vi "guadagno.vi"() -> ()   [LabVIEW 2014]
uses:
  <vilib>/measure/maspectr.llb/FFT Power Spectrum and PSD for N Chan.vi
  <vilib>/measure/mascope.llb/Amplitude and Levels N chan.vi
  <vilib>/measure/NI_MABase.lvlib
  <vilib>/measure/NI_MAPro.lvlib
panel:
  out "x/y 2":T1(array[cluster])
  out "Waveform Graph 4":cluster{"f0":dbl, "df":dbl, "magnitude":dbl[]}[](graph)
  out "x/y":dbl[](array[numeric])
  out "Waveform Graph 3":dynamicdata(graph)
  out "Waveform Graph 2":dynamicdata(graph)
  out "Waveform Graph":waveform(dbl)(graph)
  in  "signal type":T2(ring)
  in  "amplitude":dbl=1.0 format="%0.2p"
  in  "frequency":dbl=10.0 format="%#_13g"
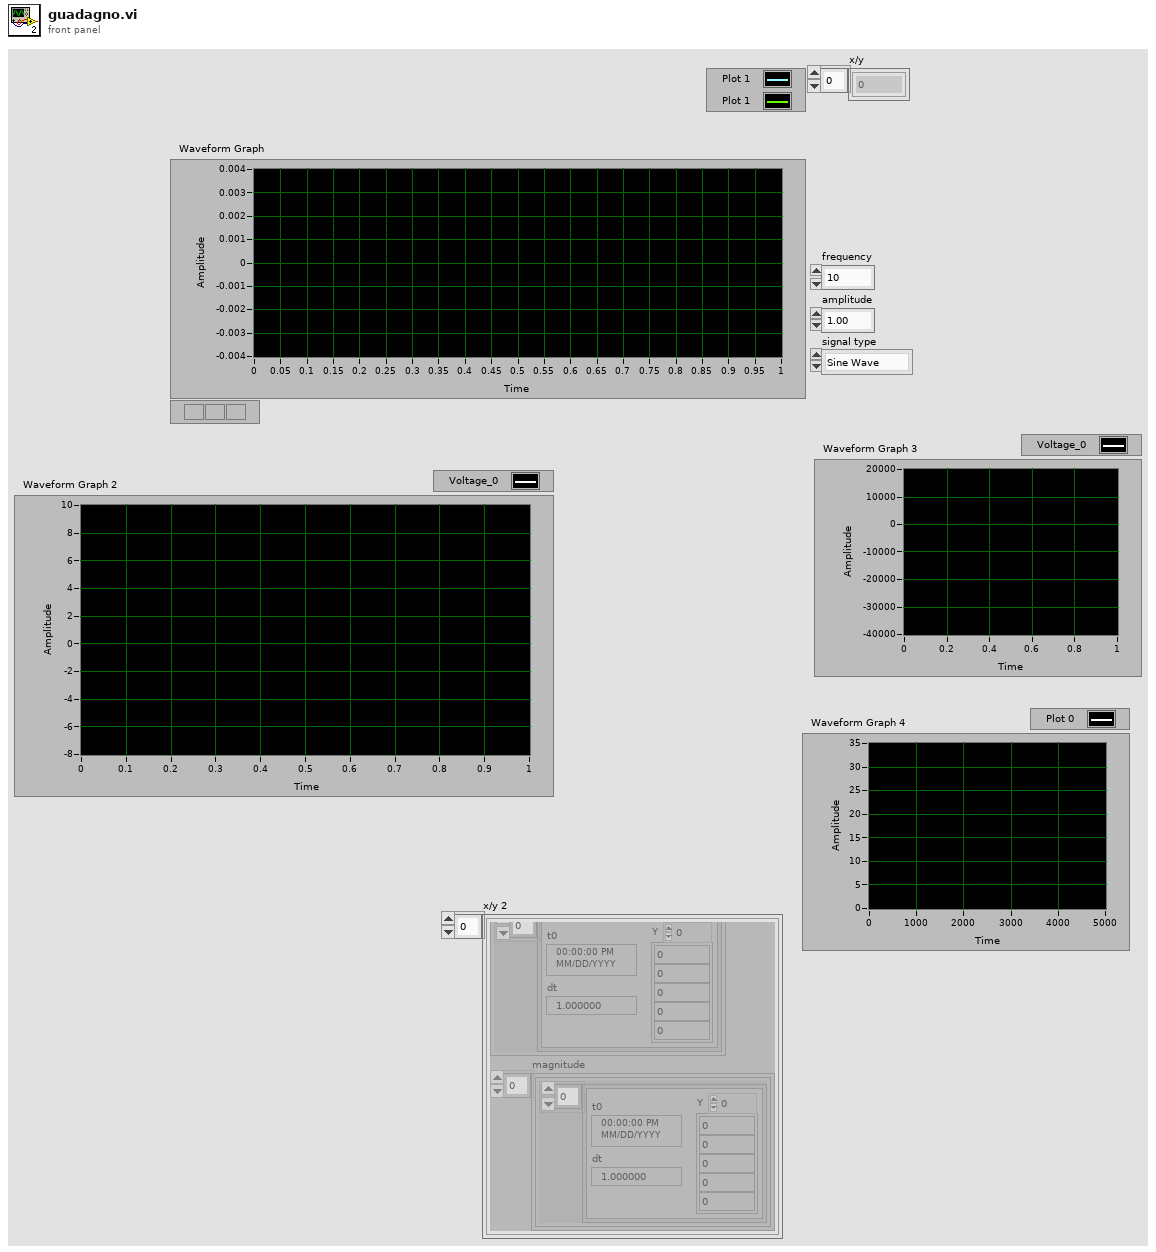
[diagram p1: front panel]
types:
  T1 = cluster{"f0":dynamicdata, "df":dynamicdata, "magnitude":dynamicdata[]}[]
  T2 = enum16{"Sine Wave", "Triangle Wave", "Square Wave", "Sawtooth Wave"}
  T3 = cluster{"method":enum32{"histogram", "peak", "auto select"}, "histogram size":i32, "histogram method":enum16{"mode"}, "reserved":dbl}
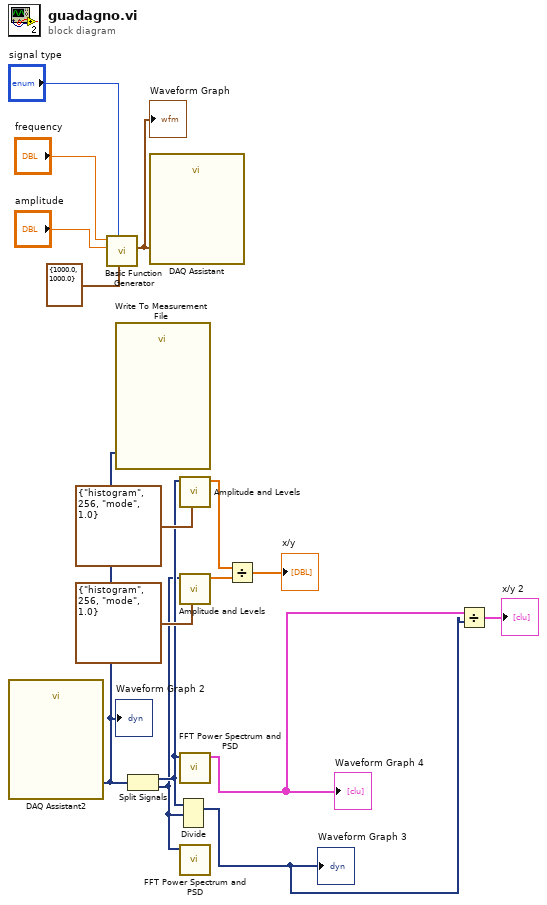
[diagram p0: block diagram]
diagram:
  n1 = call "DAQ Assistant2"() -> ("data"=w4:dynamicdata)  [unwired: 17 in, 2 out]
  "Waveform Graph 2" <- w4
  n2 = call <vilib>:"Basic Function Generator.vi"("sampling info"=cluster{"Fs":dbl, "#s":dbl} {"Fs"=1000.0, "#s"=1000.0}, "signal type"="signal type", "amplitude"="amplitude", "frequency"="frequency") -> ("signal out"=w12:waveform(dbl))  [unwired: 5 in, 2 out]
  "Waveform Graph" <- w12
  n3 = call "Write To Measurement File"("Signals"=w4) -> ()  [unwired: 16 in, 3 out]
  n4 = Split Signals(w4) -> (w6:dynamicdata, w5:dynamicdata)  [unwired: 2 in]
  n5 = call "DAQ Assistant"("data"=w12) -> ()  [unwired: 16 in, 3 out]
  n6 = Divide(1:w5, 2:w6) -> (0:w2:dynamicdata)  [unwired: 1 in, 1 out]
  "Waveform Graph 3" <- w2
  n7 = call-poly <vilib>:"Amplitude and Levels.vi"("state settings"=T3 {"method"=enum."histogram", "histogram size"=256, "histogram method"=enum."mode", "reserved"=1.0}, "signal(s) in"=w6) -> ("amplitude"=w9:dbl[])  [unwired: 6 in, 3 out]
  n8 = call-poly <vilib>:"Amplitude and Levels.vi"("state settings"=T3 {"method"=enum."histogram", "histogram size"=256, "histogram method"=enum."mode", "reserved"=1.0}, "signal(s) in"=w5) -> ("amplitude"=w8:dbl[])  [unwired: 6 in, 3 out]
  n9 = call-poly <vilib>:"FFT Power Spectrum and PSD.vi"("time signals"=w6) -> ("Power Spectrum / PSD"=w3:cluster{"f0":dbl, "df":dbl, "magnitude":dbl[]}[])  [unwired: 7 in, 3 out]
  "Waveform Graph 4" <- w3
  n10 = call-poly <vilib>:"FFT Power Spectrum and PSD.vi"("time signals"=w5) -> ()  [unwired: 7 in, 4 out]
  n11 = Divide(x=w9, y=w8) -> (x/y=→"x/y":dbl[])
  n12 = Divide(x=w3, y=w2) -> (x/y=→"x/y 2":T1)
